vi "read primary network adapter.vi"(8 "error in":errorcluster, 11 "Controller in":refnum<class "Controller.lvclass">) -> (0 "error out":errorcluster, 2 "primary network adapter":T1={"IP Address"="", "MAC Address"="", "IP Address Request Mode"=1, "SubnetMask"="", "Gateway"="", "DNS Server"="", "Adapter Mode"=1, "Adapter Type"=1} {"IP Address Request Mode" items=["Static"=1, "DHCP/Link Local"=2, "Link-Local Only"=4, "DHCP Only"=8]; "Adapter Type" items=["Ethernet"=1, "WLAN"=2]; "Adapter Mode" items=["Disabled"=1, "TCP/IP Ethernet"=2, "Deterministic"=4, "EtherCAT"=8, "TCP/IP WLAN Connect"=32, "TCP/IP WLAN Create"=64]}, 3 "Controller out":refnum<class "Controller.lvclass">)   [LabVIEW 2016, in "SMI.lvlib" / "Controller.lvclass"]
uses:
  Controller.lvclass
  NetworkAdapterSettings.ctl
  Controller.lvclass/Controller.ctl
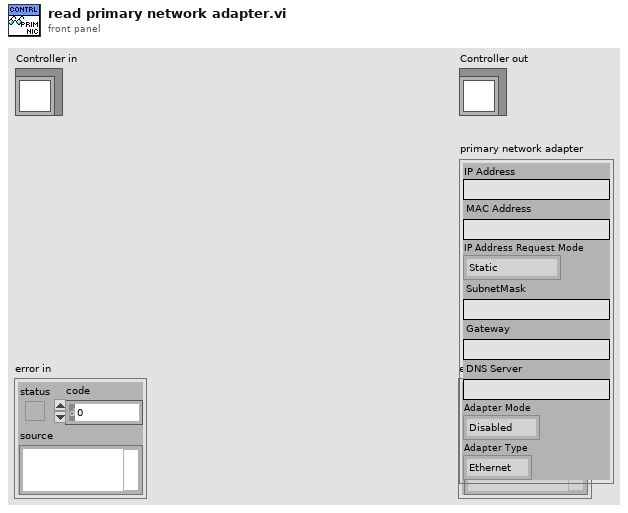
[diagram p1: front panel]
types:
  T1 = typedef "SMI.lvlib/Controller.lvclass/NetworkAdapterSettings.ctl" = cluster{"IP Address":string, "MAC Address":string, "IP Address Request Mode":u32, "SubnetMask":string, "Gateway":string, "DNS Server":string, "Adapter Mode":u32, "Adapter Type":u32}
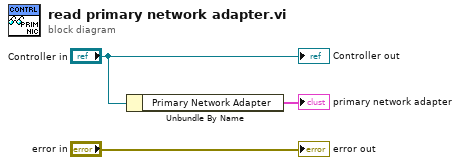
[diagram p0: block diagram]
diagram:
  n1 = Unbundle By Name("Controller in") -> ("Primary Network Adapter"=→"primary network adapter":T1)
  "error out" <- "error in"
  "Controller out" <- "Controller in"
